vi "QCA - DUT Open TCP Dll.vi"(9 "Timeout (2500ms)":i32=2500, 10 "port (2390)":u32=2390, 11 "IP Address (\"\": localhost)":string) -> (2 "StatusIsFalse":i32, 3 "NART TCP Connection":refnum<k5>)   [LabVIEW 2011]
panel:
  out "Error out with context":errorcluster
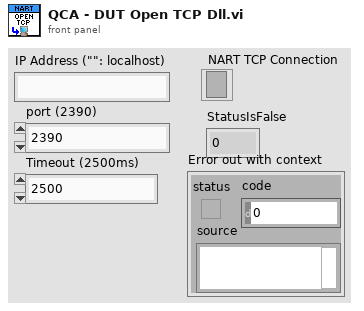
[diagram p1: front panel]
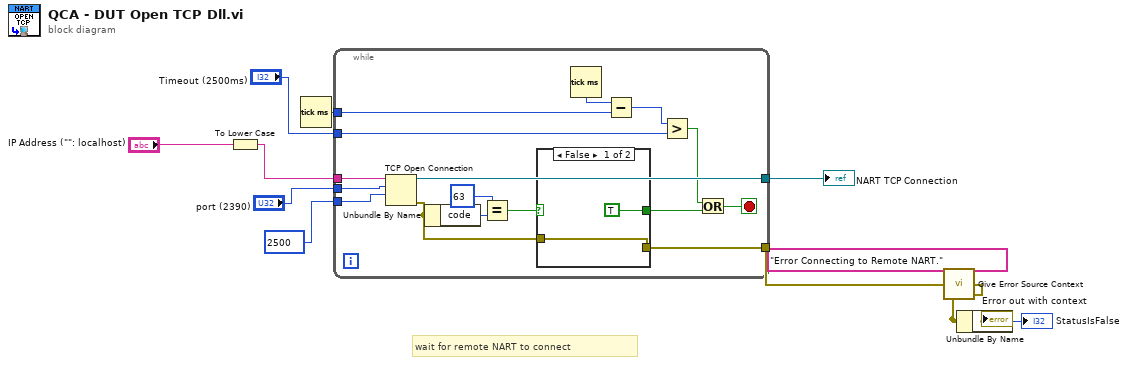
[diagram p0: block diagram]
diagram:
  # "wait for remote NART to connect"
  n1 = To Lower Case(string="IP Address (\"\": localhost)") -> (all lower case string=w4:string)
  n2 = Tick Count (ms)() -> (millisecond timer value=w9:u32)
  n3 = while {
    tunnel: [w27] -> w1
    tunnel: [w24] -> w11
    tunnel: w9 -> [w20]
    tunnel: 2500 ("timeout ms (60000)") -> [w15]
    tunnel: w4 -> [w14]
    tunnel: "port (2390)" -> [w13]
    tunnel: "Timeout (2500ms)" -> [w12]
    stop <- w16 stop-if-true
    n4 = TCP Open Connection(address=w14, remote port or service name=w13, timeout ms (60000)=w15) -> (connection ID=w27:refnum<k5>, error out=w23:errorcluster)  [unwired: 2 in]
    n5 = Unbundle By Name(w23) -> ("code"=w26:i32)
    n6 = Equal?(x=63, y=w26) -> (x = y?=w22:bool)
    n7 = case shown="False" w22 {
      tunnel: [w29 w30] -> w24
      tunnel: w23 -> [w29 w30]
      tunnel: [TRUE ("status") _] -> w17
      frame False {
      }
      frame True {
      }
    }
    n8 = Tick Count (ms)() -> (millisecond timer value=w21:u32)
    n9 = Subtract(x=w21, y=w20) -> (x-y=w19:u32)
    n10 = Greater?(x=w19, y=w12) -> (0:w18:bool)
    n11 = Or(x=w18, y=w17) -> (x .or. y?=w16:bool)
  }
  "NART TCP Connection" <- w1
  n12 = call "Give Error Source Context.vi"("Context String"="Error Connecting to Remote NART." ("string"), "error in"=w11) -> ("Error out with context"=w6:errorcluster)  [unwired: 13 in]
  "Error out with context" <- w6
  n13 = Unbundle By Name(w6) -> ("code"=→"StatusIsFalse":i32)
